vi "Initialize DataBase.vi"() -> ()   [LabVIEW 2024]
panel:
  out "DB Connected?":bool
  out "Db Path":string
  out "error out":errorcluster
  in  "error in":errorcluster
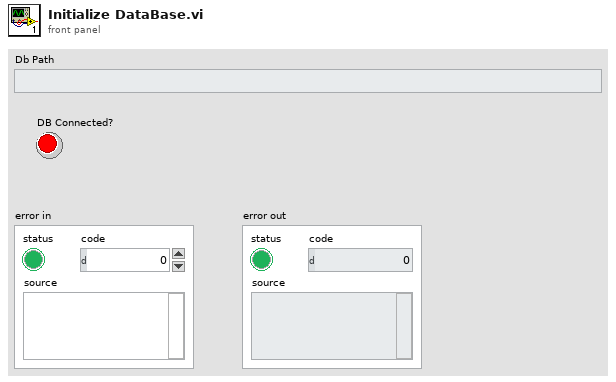
[diagram p1: front panel]
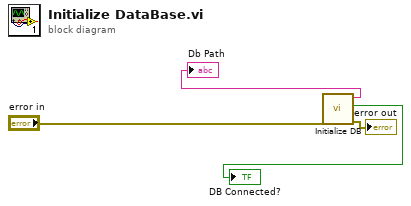
[diagram p0: block diagram]
diagram:
  n1 = call "Initialize DB.vi"("error in (no error)"="error in") -> ("error out"=→"error out":errorcluster, "DB Connected?"=→"DB Connected?":bool, "Db Path"=→"Db Path":string)  [unwired: 8 in]
